vi "WLAN DUT Update Payload Length.vi"(8 "error in (no error)":errorcluster, 11 "niDTS WLAN DUT in":refnum<class "niDTS WLAN Dut.lvclass">) -> (0 "error out":errorcluster, 3 "niDTS WLAN DUT out":refnum<class "niDTS WLAN Dut.lvclass">)   [LabVIEW 2015, in "niDTS WLAN.lvlib" / "niDTS WLAN Dut.lvclass"]
doc: "Updates the payload length to comply with DUT settings. If 16 symbols is set to TRUE, this sets the payload length according to the Standard, Rate, Streams, and Bandwidth. If 16 symbols is FALSE, the payload length is not modified. In both cases, the actual payload length is coerced by Payload Length Limit if required."
uses:
  niDTS WLAN Dut.lvclass
  niDTS WLAN Dut.lvclass/niDTS WLAN Dut.ctl
  niDTS WLAN.lvlib
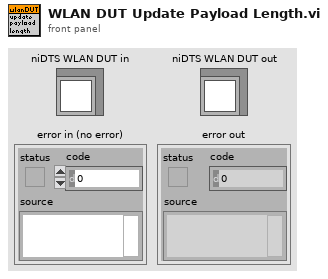
[diagram p1: front panel]
types:
  T1 = typedef "niDTS WLAN.lvlib/niDTS WLAN INC Standard.ctl" = enum16{"802.11 b DSSS", "802.11 a/g OFDM", "802.11 n HT", "802.11 ac VHT"}
  T2 = typedef "niDTS WLAN.lvlib/niDTS WLAN INC DSSS Data Rate.ctl" = enum16{"1", "2", "5.5", "11"}
  T3 = typedef "niDTS WLAN.lvlib/niDTS WLAN INC OFDM Data Rate.ctl" = enum16{"6", "9", "12", "18", "24", "36", "48", "54"}
  T4 = typedef "niDTS WLAN.lvlib/niDTS WLAN INC CH BW.ctl" = enum16{"20 MHz", "40 MHz", "80 MHz", "160 MHz"}
  T5 = typedef "niDTS WLAN.lvlib/niDTS WLAN INC Type.ctl" = enum16{"b - 1 Mbps", "b - 2 Mbps", "b - 5.5 Mbps", "b - 11 Mbps", "ag - 6 Mbps", "ag - 9 Mbps", "ag - 12 Mbps", "ag - 18 Mbps", "ag - 24 Mbps", "ag - 36 Mbps", "ag - 48 Mbps", "ag - 54 Mbps", "n - MCS0", "n - MCS1", "n - MCS2", "n - MCS3", "n - MCS4", "n - MCS5", "n - MCS6", "n - MCS7", "n - MCS8", "n - MCS9", "n - MCS10", "n - MCS11", "n - MCS12", "n - MCS13", "n - MCS14", "n - MCS15", "n - MCS16", "n - MCS17", "n - MCS18", "n - MCS19", "n - MCS20", "n - MCS21", "n - MCS22", "n - MCS23", "n - MCS24", "n - MCS25", "n - MCS26", "n - MCS27", "n - MCS28", "n - MCS29", "n - MCS30", "n - MCS31", "ac - MCS0 -1", "ac - MCS1 -1", "ac - MCS2 -1", "ac - MCS3 -1", "ac - MCS4 -1", "ac - MCS5 -1", "ac - MCS6 -1", "ac - MCS7 -1", "ac - MCS8 -1", "ac - MCS9 -1", "ac - MCS0 -2", "ac - MCS1 -2", "ac - MCS2 -2", "ac - MCS3 -2", "ac - MCS4 -2", "ac - MCS5 -2", "ac - MCS6 -2", "ac - MCS7 -2", "ac - MCS8 -2", "ac - MCS9 -2", "ac - MCS0 -3", "ac - MCS1 -3", "ac - MCS2 -3", "ac - MCS3 -3", "ac - MCS4 -3", "ac - MCS5 -3", "ac - MCS6 -3", "ac - MCS7 -3", "ac - MCS8 -3", "ac - MCS9 -3", "ac - MCS0 -4", "ac - MCS1 -4", "ac - MCS2 -4", "ac - MCS3 -4", "ac - MCS4 -4", "ac - MCS5 -4", "ac - MCS6 -4", "ac - MCS7 -4", "ac - MCS8 -4", "ac - MCS9 -4"}
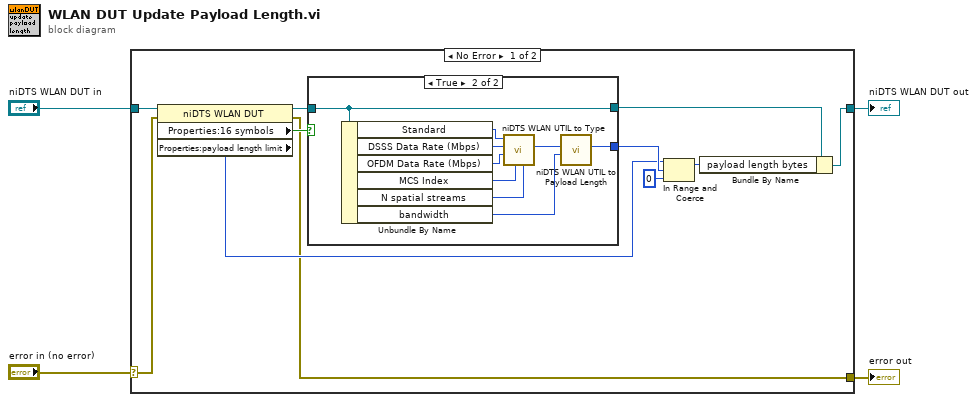
[diagram p0: block diagram]
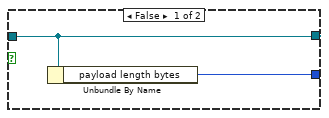
[diagram p2: hidden frame]
diagram:
  n1 = case shown="No Error" "error in (no error)" {
    selector: "error in (no error)" -> [w12 w28]
    tunnel: [w5 w28] -> w3
    tunnel: [w6 w27] -> w1
    tunnel: "niDTS WLAN DUT in" -> [w15 w27]
    frame No Error {
      n2 = property class="niDTS WLAN DUT"(reference=w15, error in=w12) -> (reference out=w13:refnum<class "niDTS WLAN Dut.lvclass">, error out=w5:errorcluster, "Properties:16 symbols"=w14:bool, "Properties:payload length limit"=w9:i32)
      n3 = case shown="True" w14 {
        tunnel: w13 -> [w16 w19]
        tunnel: [w16 w19] -> w8
        tunnel: [w17 w18] -> w10
        frame False {
          n4 = Unbundle By Name(w16) -> ("payload length bytes"=w17:i32)
        }
        frame True {
          n5 = Unbundle By Name(w19) -> ("Standard"=w26:T1, "DSSS Data Rate (Mbps)"=w25:T2, "OFDM Data Rate (Mbps)"=w24:T3, "MCS Index"=w23:i32, "N spatial streams"=w22:i32, "bandwidth"=w20:T4)
          n6 = call "niDTS WLAN UTIL to Type.vi"("N_SS"=w22, "MCS"=w23, "OFDM Data Rate (Mbps)"=w24, "DSSS Data Rate (Mbps)"=w25, "Standard"=w26) -> ("WLAN Type"=w21:T5)  [unwired: 6 in]
          n7 = call "niDTS WLAN UTIL to Payload Length.vi"("CH BW"=w20, "WLAN Type"=w21) -> ("Payload Length"=w18:i32)  [unwired: 9 in]
        }
      }
      n8 = In Range and Coerce(upper limit=w9, x=w10, lower limit=0) -> (coerced(x)=w7:i32)  [unwired: 1 out]
      n9 = Bundle By Name(cluster=w8, "payload length bytes"=w7) -> (w6:refnum<class "niDTS WLAN Dut.lvclass">)
    }
    frame Error {
    }
  }
  "error out" <- w3
  "niDTS WLAN DUT out" <- w1
